vi "FestoCPX.Station.Table.Rotate.vi"(6 "Timeout [ms] (7500)":i32=5000, 8 "error in":errorcluster) -> (0 "error out":errorcluster)   [LabVIEW 2016]
uses:
  Station/Station.ValvePosition.ctl
  tools/EventLog/EventLog.EventSource.ctl
  tools/Translator/Translator.Message.ctl
  tools/EventLog/EventLog.CreateError(array).vi
  tools/Translator/Translator.Translate.Status (NoError).vi
  tools/Translator/Translator.FormatMessage.vi
  Station/Station.Global.vi
  tools/Translator/Translator.Global.vi
  tools/ErrorHandling/ErrorHandling.Create.vi
panel:
  out "rotated?":bool
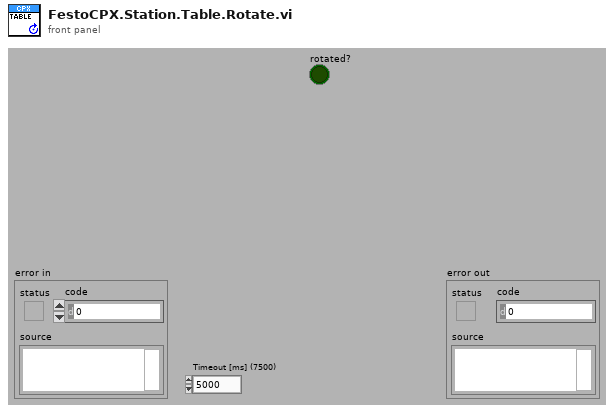
[diagram p1: front panel]
types:
  T1 = typedef "Station.ValvePosition.ctl" = enum16{"Home", "Work"}
  T2 = typedef "Translator.Message.ctl" = enum16{"-", "Event confirmed", "Log out", "Log in", "Shutdown", "Cancel", "Start", "Begin time", "End time", "Duration", "Service Mode", "Ignore Results", "Serial Format", "On", "Off", "OK", "NOK", "NOK %s", "Home", "Work", "Close", "Open", "In progress...", "Missing", "Empty", "Hardware failure", "Initial", "Default", "Total", "Out of range", "Free disk space is below 1GB - contact technician", "Error %d >> %s", "Error %d >> %s >> %s", "Msg %d >> %s", "Laser msg %d %s", "Laser cmd error %s %d", "Laser cmd failed %s", "Laser cmd warning %s", "Laser disconnected", "Laser status %s", "Laser already started", "Laser job unkonwn %s", "Laser job missing %s", "Laser job select failure %s", "Unable to start laser printing (%s)", "Unable to stop laser printing (%s)", "Laser marking aborted", "Laser marking timeout", "Unable to reset Laser Interlock (%s)", "Unable to trigger Laser. Laser not ready (%s)", "Laser job '%s' coordinates not configured", "Starting %s", "Quitting %s", "Configured", "Initializing", "Quitting", "Loading", "Loaded %d results", "Loaded %d events", "Running", "Stopped", "Summary", "Laser", "Do you want to continue?", "Do you want to delete the configuration?", "The configuration is being used by an order. Unable to delete!", "Press confirm button", "Station is not based. Do you want to exit?", "Station requires changeover. Do you want to run the test?", "Test options are not set as default. Do you want to continue?", "Formatting of WabcoNo is disabled. Do you want to continue?", "Product not detected. Do you want to continue?", "Product scan failed. Do you want to continue?", "Calibration", "Log out?", "System", "All", "IDLE", "Translating...%s", "Not found", "Alarm %s", "Run", "Skip", "Abort", "Repeat", "Please wait...", "Database disconnected", "Database disconnected - changeover disabled!", "Login to database successful", "Login to database failed: %d; %s", "Unable to check the product status of reference %d - database disconnected", "Unable to set the product status of reference %d - database disconnected", "Variant file backup %s", "Read variant (%s)", "Result", "Station armed!", "Station requires changeover!", "Select reference number...", "EMERGENCY BUTTON - press Control button", "EMERGENCY DOOR - press Control button", "Resetting Emergency...", "Unable to reset safety circuit - Emergency Button pressed", "Unable to reset safety circuit - Emergency Side Door open", "Station not based", "Station based", "Station not empty", "Station basing...", "No order", "Press Start to begin new order", "Scanning new order", "Order NOK. Correct or scan again", "Order OK. Press Accept", "Order ready", "Revolver incorrect", "Fork incorrect", "Revolver missing", "Revolver empty", "Container missing", "Offline results", "Offline statistics", "Updating statistics %.1f %%", "DMC Configurator", "Door open", "Close the front door", "Press start button", "Done. Open the front door", "Running...", "Running...%.1f %%", "Pause %s", "Pause %s. NOK container missing", "Pause %s. OK container missing", "Pause %s. Revolver empty", "Pause %s. Revolver missing", "Pause %s. Revolver incorrect", "Pause %s. Fork missing", "Pause %s. Fork incorrect", "Pause %s. Too many failures", "Pause %s. Unloading failure", "Pause %s. One slot is not working", "Pause %s. Part order is done. Empty OK container", "Pause %s. Unable to move product to slot", "Pause %s. Unable to move back product pusher", "Pause %s. Unable to lift product", "Pause %s. Unable to move back product lifter", "Pause %s. Unable to move product arm to Work", "Pause %s. Unable to move product arm to NOK", "Pause %s. Unable to move product arm to OK", "Pause %s. Unable to unsuck the NOK product", "Pause %s. Unable to drop the NOK product", "Pause %s. Product OK missing", "Pause %s. Unable to unsuck the OK product", "Pause %s. Unable to drop the OK product", "Stopping...", "File '%s' is missing", "File '%s' is broken", "File '%s' is running", "Log file started (%s)", "Log file ended (%s)", "Log file stopped (%s)", "Log file ignored (%s)", "Log file exported (%s)", "Log file export failed (%s)", "Wrong serial number in log file", "Wrong reference number in log file", "Test steps are missing", "%s = %.3f", "Process param '%s' not found in DB", "Process param '%s' wrong order", "Process param '%s' value %.3f out of limits (%.3f; %.3f)", "Step%d param '%s' not found in DB", "Step%d param '%s' wrong order", "Step%d param '%s' value %.3f out of limits (%.3f; %.3f)", "Step%d EV '%s' not found in DB", "Step%d EV '%s' wrong order", "\"%s\" not found in DB", "\"%s\" wrong order", "\"%s\" value %.3f out of limits (%.3f; %.3f)", "\"%s\" not found in software", "Process init (%s)", "Process started", "Process restarted", "Process run", "Process done", "Process done - remove OK container", "Process aborted", "Process aborted at work", "Process aborted at home", "Process error", "Process error at home", "Process error at work", "Process close", "Process pause", "Process continue", "Process door open", "Process door close", "Process pause at slot %s due to %s", "Select plate from the order to process", "Do you want to start the process?", "Do you want to continue the process?", "There is unfinished order. Do you want to put the new order?", "Product %s %d OK", "Product %s %d NOK", "Unable to unload the slot %s. Product missing in the slot", "Unable to unload the slot %s. Product already in the arm", "Unable to accept the product as OK. Product missing in slot %s", "Unable to accept the product as OK. Product could not drop into the container at slot %s", "Unable to accept the product as NOK. Product could not drop into the container at slot %s", "Scan failed. Error %s", "Scan failed. Scanner disconnected", "Scan failed. Wrong Wabco number %d, limit (%d,%d)", "Scan failed. Wrong serial number %d, limit (%d,%d)", "Scan failed. Wrong date %d, limit (%d,%d)", "Scan failed. Wrong product wabco number %d (expected %d)", "Scan failed. Wrong product serial number %d (expected > 0)", "Scan OK %s", "Scan failed. Unable to determine table position (%s)", "Scan failed. Timeout", "Tune failed. Scanner disconnected", "Tune failed. Timeout", "%s = %d", "%s = %d->%d", "Unable to set %s = %.2f - Air Pressure Inside off", "Unable to set digital output '%s' = %d", "Unable to activate air pressure inside - timeout", "Unable to activate air pressure inside - aborted", "Unable to switch on Air Main Valve - Air Pressure Inlet off", "Unable to switch on Air Main Valve - Door open", "Unable to switch off Air Main Valve - timeout", "Unable to switch off Air Main Valve - aborted", "Unable to rotate Table - timeout", "Unable to rotate Table - aborted", "Unable to rotate Table - Product Move not in Home position", "Unable to rotate Table - Air Pressure Inside off", "Unable to rotate Table - Product Lift A not in Home position", "Unable to rotate Table - Product Lift B not in Home position", "Unable to rotate Table - unlock before movement timeout", "Unable to rotate Table - lock after movement timeout", "Unable to move Table Lock to %s position - timeout", "Unable to move Table Lock to %s position - aborted", "Unable to move Table Lock to %s position - Air Pressure Inside off", "Unable to move Table Lock to %s position - Table not in position", "Unable to move Product Lift A to %s position - timeout", "Unable to move Product Lift B to %s position - timeout", "Unable to move Product Lift A to %s position - aborted", "Unable to move Product Lift B to %s position - aborted", "Unable to move Product Lift A to %s position - Air Pressure Inside off", "Unable to move Product Lift B to %s position - Air Pressure Inside off", "Unable to move Product Lift A to %s position - Table not locked", "Unable to move Product Lift B to %s position - Table not locked", "Unable to move Product Lift A to %s position - Product Arm not in Work position", "Unable to move Product Lift B to %s position - Product Arm not in Work position", "Unable to set Product Suction Gripper %s to %s - timeout", "Unable to set Product Suction Gripper %s to %s - aborted", "Unable to set Product Suction Gripper %s to %s - Air Pressure Inside off", "Unable to set Product Suction Gripper %s to %s - Table slot unkown", "Unable to move Product Arm to %s position - timeout", "Unable to move Product Arm to %s position - aborted", "Unable to move Product Arm to %s position - Air Pressure Inside off", "Unable to move Product Arm to %s position - Product Lift A not in Home position", "Unable to move Product Arm to %s position - Product Lift B not in Home position", "Unable to move Product to %s position - timeout", "Unable to move Product to %s position - aborted", "Unable to move Product to %s position - Air Pressure Inside off", "Unable to move Product to %s position - Table not in position"}
  T3 = typedef "EventLog.EventSource.ctl" = enum16{"All", "Gui", "Ref", "File", "Arch", "Seq", "CPX", "DB", "Laser", "Scan.P", "Scan.O"}
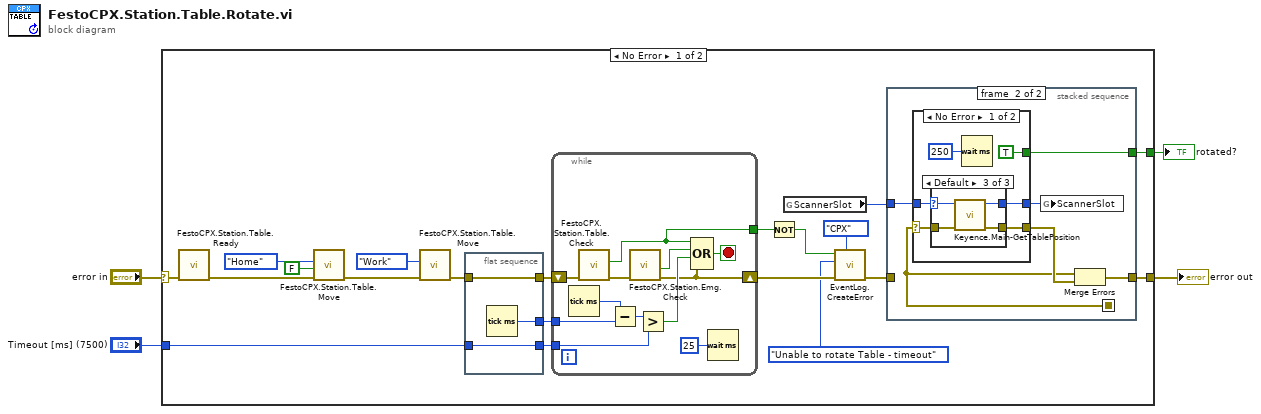
[diagram p0: block diagram]
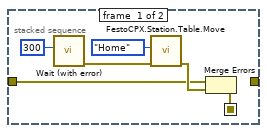
[diagram p2: hidden frame]
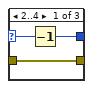
[diagram p3: hidden frame]
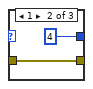
[diagram p4: hidden frame]
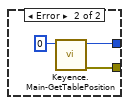
[diagram p5: hidden frame]
diagram:
  n1 = case shown="No Error" "error in" {
    selector: "error in" -> [w24 w70]
    tunnel: [w23 w70] -> w4
    tunnel: "Timeout [ms] (7500)" -> [w22 _]
    tunnel: [w5 _] -> w1
    frame No Error {
      n2 = call "FestoCPX.Station.Table.Ready.vi"("error in"=w24) -> ("error out"=w6:errorcluster)  [unwired: 9 in, 1 out]
      n3 = call "FestoCPX.Station.Table.Move.vi"("error in"=w6, "Wait for input signal? (T)"=FALSE, "Position"=Station.ValvePosition."Home") -> ("error out"=w12:errorcluster)  [unwired: 8 in]
      n4 = call "FestoCPX.Station.Table.Move.vi"("error in"=w12, "Position"=Station.ValvePosition."Work") -> ("error out"=w11:errorcluster)  [unwired: 9 in]
      n5 = flat-sequence {
        tunnel: w11 -> [w57]
        tunnel: [w57] -> w21
        tunnel: [w56] -> w20
        tunnel: [w55] -> w9
        tunnel: w22 -> [w55]
        frame #0 {
          n6 = Tick Count (ms)() -> (millisecond timer value=w56:u32)
        }
      }
      n7 = while {
        shift-right: [w60] -> w18
        shift-left: w21 -> [w69]
        tunnel: w20 -> [w67]
        tunnel: w9 -> [w65]
        tunnel: [w58] -> w17
        stop <- w64 stop-if-true
        n8 = Tick Count (ms)() -> (millisecond timer value=w68:u32)
        n9 = call "FestoCPX.Station.Table.Check.vi"("error in"=w69) -> ("error out"=w61:errorcluster, "Table Pos"=w58:bool)  [unwired: 8 in, 1 out]
        n10 = Subtract(x=w68, y=w67) -> (x-y=w66:u32)
        n11 = call "FestoCPX.Station.Emg.Check.vi"("error in"=w61) -> ("error out"=w60:errorcluster, "Emg occured"=w59:bool)  [unwired: 8 in, 1 out]
        n12 = Greater?(x=w66, y=w65) -> (0:w62:bool)
        n13 = Compound Arithmetic op=OR(w58, w59, w62, w60) -> (w64:bool)
        n14 = Wait (ms)(milliseconds to wait=u32 25) -> ()  [unwired: 1 out]
      }
      n15 = Not(x=w17) -> (.not. x?=w16:bool)
      n16 = global read "Station.Global.vi" "ScannerSlot"() -> (w7:i32)
      n17 = call-poly "EventLog.CreateError.vi"("Source (All)"=EventLog.EventSource."CPX", "error in"=w18, "msg"=Translator.Message."Unable to rotate Table - timeout", "create (T)"=w16) -> ("error out"=w8:errorcluster)  [unwired: 6 in, 1 out]
      n18 = stacked-sequence {
        seq-local: [w25 _] -> [_ w32]
        tunnel: w8 -> [w26 _]
        tunnel: [_ w35] -> w23
        tunnel: w7 -> [_ w36]
        tunnel: [_ w31] -> w5
        frame #0 {
          n19 = call "Wait (with error).vi"("milliseconds to wait"=u32 300) -> ("error out"=w29:errorcluster)  [unwired: 9 in, 1 out]
          n20 = call "FestoCPX.Station.Table.Move.vi"("error in"=w29, "Position"=Station.ValvePosition."Home") -> ("error out"=w27:errorcluster)  [unwired: 9 in]
          n21 = Merge Errors(w26, w27) -> (w25:errorcluster)
        }
        frame #1 {
          n22 = case shown="No Error" w32 {
            selector: w32 -> [w40 _]
            tunnel: w36 -> [w42 _]
            tunnel: [w41 w53] -> w33
            tunnel: [w39 w54] -> w34
            tunnel: [TRUE _] -> w31
            frame No Error {
              n23 = case shown="Default" w42 {
                selector: w42 -> [w45 _ w49]
                tunnel: [w44 4 w48] -> w41
                tunnel: w40 -> [w43 w46 w51]
                tunnel: [w43 w46 w50] -> w39
                frame 2..4 {
                  n24 = Decrement(x=w45) -> (x-1=w44:i32)
                }
                frame 1 {
                }
                frame Default {
                  n25 = call "Keyence.Main-GetTablePosition.vi"("error in (no error)"=w51, "ScannerSlot in"=w49) -> ("error out"=w50:errorcluster, "ScannerSlot out"=w48:i32)  [unwired: 7 in, 1 out]
                }
              }
              n26 = Wait (ms)(milliseconds to wait=u32 250) -> ()  [unwired: 1 out]
            }
            frame Error {
              n27 = call "Keyence.Main-GetTablePosition.vi"("ScannerSlot in"=0) -> ("error out"=w54:errorcluster, "ScannerSlot out"=w53:i32)  [unwired: 8 in, 1 out]
            }
          }
          n28 = global write "Station.Global.vi" "ScannerSlot"(w33) -> ()
          n29 = Merge Errors(w32, w34) -> (w35:errorcluster)
        }
      }
    }
    frame Error {
    }
  }
  "error out" <- w4
  "rotated?" <- w1
